vi "Add Points.vi"(8 "error in (no error)":errorcluster, 10 "Solid Lines":i32[](array[numeric]), 11 "Game Engine in":refnum<class "Game Engine.lvclass">) -> (0 "error out":errorcluster, 2 "Solid Lines (duplicate)":i32[](array[numeric]), 3 "Game Engine out":refnum<class "Game Engine.lvclass">)   [LabVIEW 2017, in "Game Engine.lvlib" / "Game Engine.lvclass"]
uses:
  Game Engine.lvclass
  Game Engine.lvclass/Game Engine.ctl
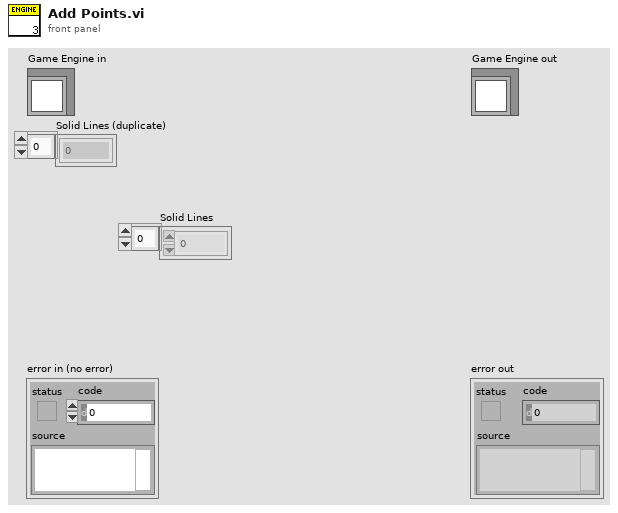
[diagram p1: front panel]
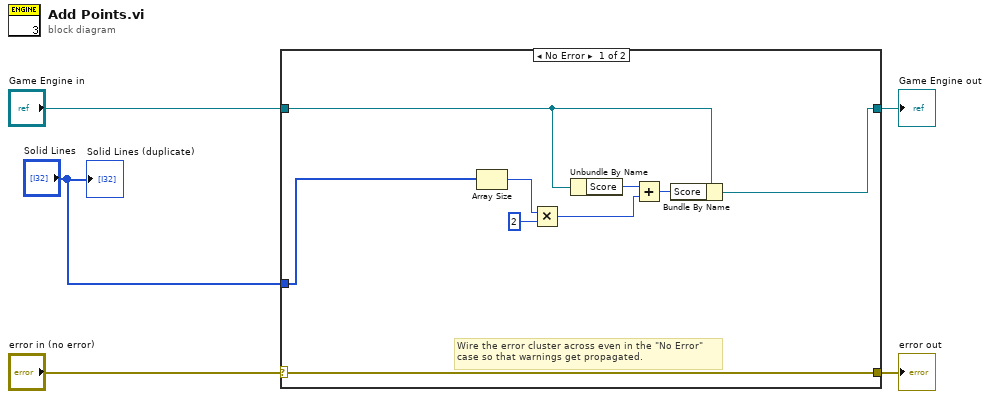
[diagram p0: block diagram]
diagram:
  n1 = case shown="No Error" "error in (no error)" {
    selector: "error in (no error)" -> [w14 w16]
    tunnel: [w14 w16] -> w4
    tunnel: [w7 w15] -> w2
    tunnel: "Game Engine in" -> [w8 w15]
    tunnel: "Solid Lines" -> [w6 _]
    frame No Error {
      # "Wire the error cluster across even in the \"No Error\"\ncase so that warnings get propagated."
      n2 = Array Size(array=w6) -> (size(s)=w13:i32)
      n3 = Multiply(x=w13, y=2) -> (x*y=w10:i32)
      n4 = Unbundle By Name(w8) -> ("Score"=w11:u32)
      n5 = Add(x=w11, y=w10) -> (x+y=w9:u32)
      n6 = Bundle By Name(cluster=w8, "Score"=w9) -> (w7:refnum<class "Game Engine.lvclass">)
    }
    frame Error {
    }
  }
  "error out" <- w4
  "Game Engine out" <- w2
  "Solid Lines (duplicate)" <- "Solid Lines"
